vi "addFileCategory.vi"(1 "VarableID":T1) -> ()   [LabVIEW 2010]
uses:
  VarableID.ctl
  VarableStruct.ctl
  AmmeterGlobalCostants.vi
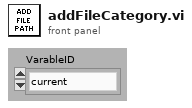
[diagram p1: front panel]
types:
  T1 = typedef "VarableID.ctl" = enum16{"current", "power", "PF", "voltage"}
  T2 = typedef "VarableStruct.ctl" = cluster{"Name":string, "StorageRefnum":refnum<file>, "Command":string, "IsDetecting":bool, "VarableID":T1}
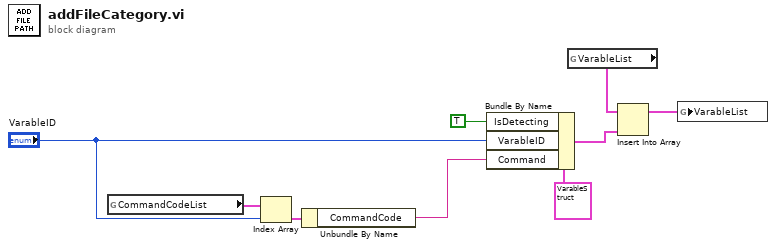
[diagram p0: block diagram]
diagram:
  n1 = global read "AmmeterGlobalCostants.vi" "CommandCodeList"() -> (w4:cluster{"CommandCode":string, "VarableID":T1}[])
  n2 = Index Array(array=w4, index="VarableID") -> (element=w3:cluster{"CommandCode":string, "VarableID":T1})
  n3 = Unbundle By Name(w3) -> ("CommandCode"=w2:string)
  n4 = Bundle By Name(cluster=T2 {"Name"="", "StorageRefnum"=refnum, "Command"="", "IsDetecting"=FALSE, "VarableID"=enum."current"} ("element"), "IsDetecting"=TRUE, "VarableID"="VarableID", "Command"=w2) -> (w5:T2)
  n5 = global read "AmmeterGlobalCostants.vi" "VarableList"() -> (w7:T2[])
  n6 = Insert Into Array(array=w7, new element=w5) -> (w6:T2[])  [unwired: 1 in]
  n7 = global write "AmmeterGlobalCostants.vi" "VarableList"(w6) -> ()
